vi "Init Platform Plugins.vi"(8 "error in (no error)":errorcluster, 11 "App in":refnum<class "App.lvclass">) -> (0 "error out":errorcluster, 3 "App out":refnum<class "App.lvclass">)   [LabVIEW 2020, in "PicoG-App.lvlib" / "App.lvclass"]
uses:
  App.lvclass
  App.lvclass/App.ctl
  Builds/picoG/ppl/PicoG-Core.lvlibp/PicoG-Processor/PicoG-Core/PlatformPluginManager/PlatformPluginManager.lvclass
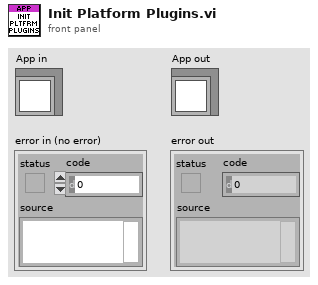
[diagram p1: front panel]
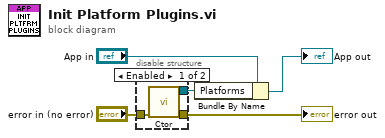
[diagram p0: block diagram]
diagram:
  n1 = disable-structure shown="Enabled" {
    disable-tunnel: [w8 _] -> w4
    disable-tunnel: "error in (no error)" -> [w7 _]
    disable-tunnel: [w6 _] -> w1
    frame Enabled {
      n2 = call "Ctor.vi"("error in (no error)"=w7) -> ("error out"=w6:errorcluster, "TargetPluginManager out"=w8:refnum<class "PlatformPluginManager.lvclass">)  [unwired: 9 in]
    }
    frame Disabled {
    }
  }
  "error out" <- w1
  n3 = Bundle By Name(cluster="App in", "Platforms"=w4) -> (→"App out":refnum<class "App.lvclass">)
